vi "Get_Notifier_REF_Once.vi"() -> (3 "notifier ref out":refnum<notifier>, 4 "notification":T1={"navX Action"=enum."Zero-Yaw", "Data"=variant, "Stream Type"=enum."YRPH", "Device Number"=enum."Dev0"})   [LabVIEW 2019]
uses:
  <vilib>/Rock Robotics/WPI/ThirdParty/Sensors/navX/_TypeDefs/Z900_navX_NotifyPacketTypeDef.ctl
  <vilib>/Rock Robotics/WPI/ThirdParty/Sensors/navX/_TypeDefs/Z900_navX_ActionTypeDef.ctl
  <vilib>/Rock Robotics/WPI/ThirdParty/Sensors/navX/_TypeDefs/Z900_navX_SerialStreamTypeDef.ctl
  <vilib>/Rock Robotics/WPI/ThirdParty/Sensors/navX/_TypeDefs/FRIC_navX_DeviceNumbersTypeDef.ctl
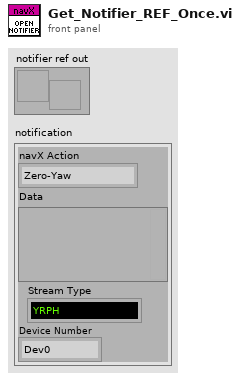
[diagram p1: front panel]
types:
  T1 = typedef "Z900_navX_NotifyPacketTypeDef.ctl" = cluster{"navX Action":T2, "Data":variant, "Stream Type":T3, "Device Number":T4}
  T2 = typedef "Z900_navX_ActionTypeDef.ctl" = enum16{"None", "Halt", "Normal Read", "Update Serial Protocol", "Update Rate Htz", "Zero-Yaw", "Zero-Displacement", "Zero-Velocity"}
  T3 = typedef "Z900_navX_SerialStreamTypeDef.ctl" = enum16{"YRPH", "Quaterinons", "Gyro/Raw", "AHRS", "AHRSAndPositioning", "AHRSAndPOSTime"}
  T4 = typedef "FRIC_navX_DeviceNumbersTypeDef.ctl" = enum16{"Dev0", "Dev1", "Dev2", "Dev3"}
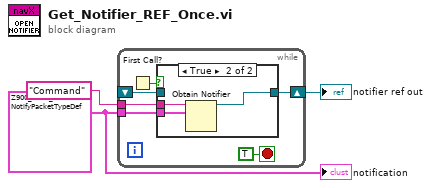
[diagram p0: block diagram]
diagram:
  w2 = T1 {"navX Action"=enum."Zero-Yaw", "Data"=variant, "Stream Type"=enum."YRPH", "Device Number"=enum."Dev0"} ("notification")
  n1 = while {
    tunnel: "Command" ("name (unnamed)") -> [w9]
    tunnel: w2 -> [w8]
    shift-right: [w5] -> w1
    shift-left: _ -> [w4]
    stop <- TRUE stop-if-true
    n2 = First Call?() -> (First Call?: T/F=w7:bool)
    n3 = case shown="True" w7 {
      tunnel: w9 -> [_ w13]
      tunnel: w8 -> [_ w12]
      tunnel: [w10 w11] -> w5
      tunnel: w4 -> [w10 _]
      frame False {
      }
      frame True {
        n4 = Obtain Notifier(name (unnamed)=w13, notification data type=w12) -> (notifier out=w11:refnum<notifier>)  [unwired: 2 in, 2 out]
      }
    }
  }
  "notifier ref out" <- w1
  "notification" <- w2
